vi "Alarm Editor.vi"() -> ()   [LabVIEW 2020]
uses:
  <vilib>/Tag Engine/Tag Expr/Tag Expr.lvclass
  C:/Program Files (x86)/National Instruments/LabVIEW 2020/vi.lib/LAVA/muParser/mupExpr/mupExpr.lvclass
  <vilib>/Tag Engine/Tag/Tag.lvclass/Tag.ctl
  cd2f347f-65b6-438d-b97c-e7d356f4cfc3.vi
  <vilib>/Tag Engine/API/Get Tag Value_ByRef.vi
  <vilib>/Tag Engine/API/Get Tag.vi
  <vilib>/Tag Engine/API/Send Tag SetRequest_ByRef.vi
  <vilib>/Tag Engine/Tag/Read Value.vi
  <vilib>/Tag Engine/Tag/Read Timestamp.vi
  <vilib>/Tag Engine/Tag/Write SetRequest.vi
  <vilib>/Tag Engine/Core/Tag Lookup_By Name.vi
  c6dfc7c3-9080-4d04-b6fb-254d10b3aea1.vi
panel:
  in  "Cancel":bool
  in  "OK":bool
  out "Name2":string
  out "Valid2":bool
  in  "Condition2":string
  out "Name1":string
  out "Valid1":bool
  in  "Condition1":string
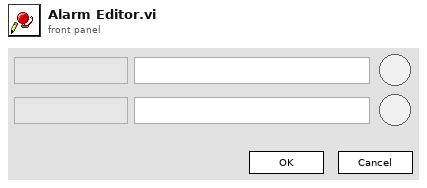
[diagram p1: front panel]
types:
  T1 = cluster{"Alarms":cluster{"Name":string, "Condition":string}[]}
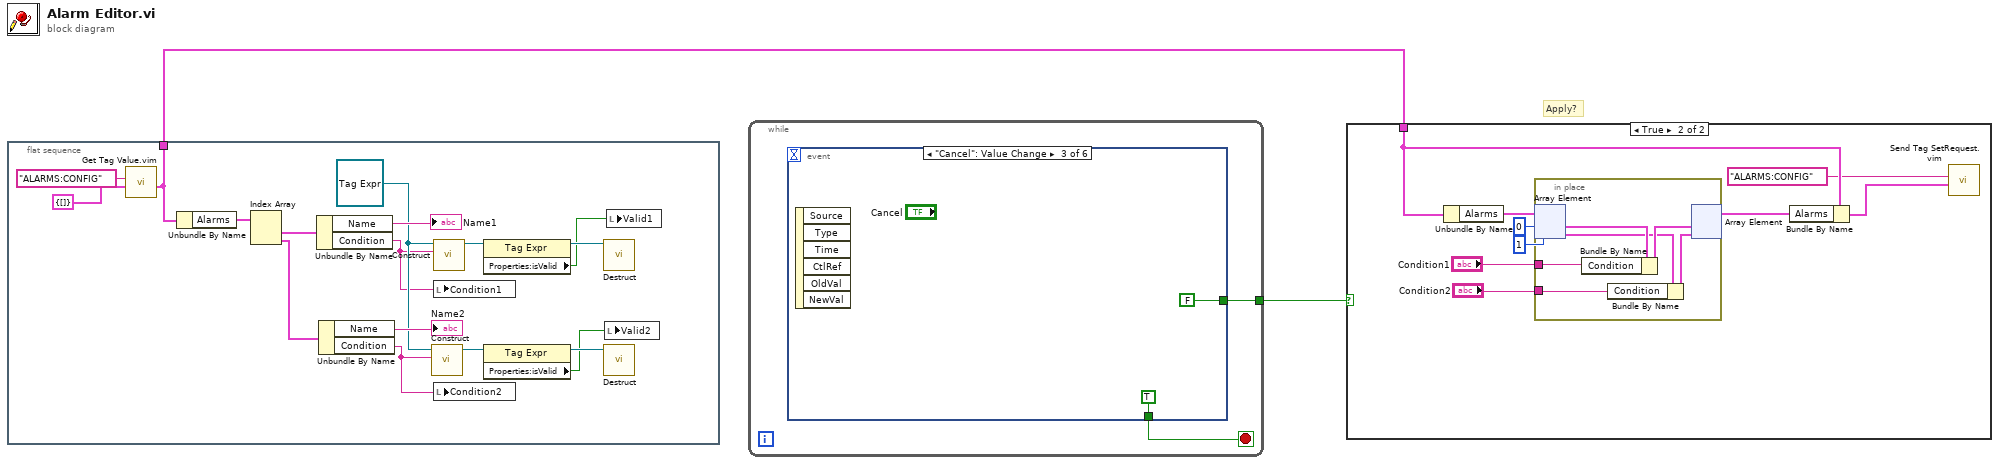
[diagram p0: block diagram]
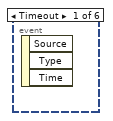
[diagram p3: hidden frame]
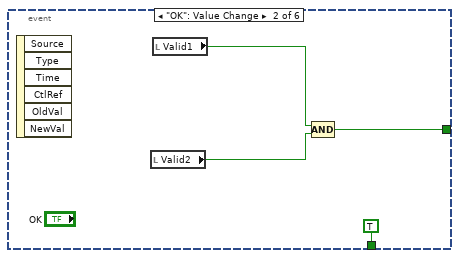
[diagram p4: hidden frame]
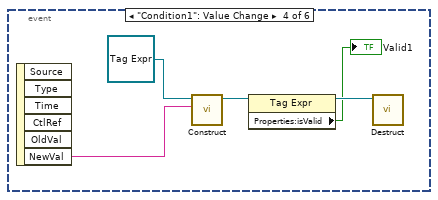
[diagram p5: hidden frame]
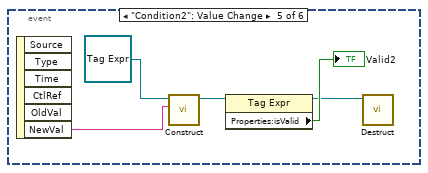
[diagram p6: hidden frame]
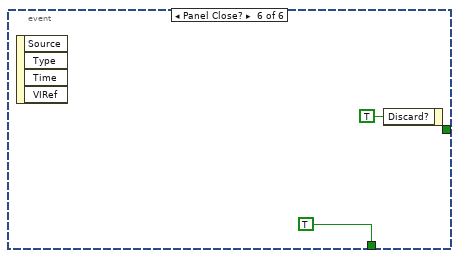
[diagram p7: hidden frame]
diagram:
  # "Apply?"
  n1 = flat-sequence {
    tunnel: [w3] -> w1
    frame #0 {
      w12 = refnum<class "Tag Expr.lvclass"> refnum ("Tag Expr in")
      n2 = call "Get Tag Value.vim"("Default (Void)"=T1 {"Alarms"=[]} ("Config"), "Tag Name(s)/Ref(s)"="ALARMS:CONFIG") -> ("Value(s)"=w3:T1)  [unwired: 6 in, 3 out]
      n3 = Unbundle By Name(w3) -> ("Alarms"=w17:cluster{"Name":string, "Condition":string}[])
      n4 = Index Array(array=w17) -> (element #1=w16:cluster{"Name":string, "Condition":string}, element #2=w14:cluster{"Name":string, "Condition":string})  [unwired: 2 in]
      n5 = Unbundle By Name(w16) -> ("Name"=→"Name1":string, "Condition"=w4:string)
      n6 = Unbundle By Name(w14) -> ("Name"=→"Name2":string, "Condition"=w5:string)
      n7 = call-dynamic "Construct.vi"("Expression"=w5, "Tag Expr in"=w12) -> ("Tag Expr out"=w10:refnum<class "Tag Expr.lvclass">)  [unwired: 6 in, 3 out]
      n8 = call-dynamic "Construct.vi"("Expression"=w4, "Tag Expr in"=w12) -> ("Tag Expr out"=w11:refnum<class "Tag Expr.lvclass">)  [unwired: 6 in, 3 out]
      n9 = local write "Condition1"(w4) -> ()
      n10 = local write "Condition2"(w5) -> ()
      n11 = property class="Tag Expr"(reference=w11) -> (reference out=w9:refnum<class "Tag Expr.lvclass">, "Properties:isValid"=w7:bool)  [unwired: 1 in, 1 out]
      n12 = property class="Tag Expr"(reference=w10) -> (reference out=w8:refnum<class "Tag Expr.lvclass">, "Properties:isValid"=w6:bool)  [unwired: 1 in, 1 out]
      n13 = call-dynamic "Destruct.vi"("muExpr in"=w9) -> ()  [unwired: 10 in, 1 out]
      n14 = call-dynamic "Destruct.vi"("muExpr in"=w8) -> ()  [unwired: 10 in, 1 out]
      n15 = local write "Valid2"(w6) -> ()
      n16 = local write "Valid1"(w7) -> ()
    }
  }
  n17 = while {
    tunnel: [w20] -> w2
    stop <- w21 stop-if-true
    n18 = event shown="[2] \"Cancel\": Value Change" {
      selector: _ -> [_ _ _ _ _ _]
      dyn-events: _ -> [_ _ _ _ _ _]
      timeout: _ -> [_ _ _ _ _ _]
      tunnel: [_ TRUE TRUE _ _ TRUE] -> w21
      tunnel: [_ w23 FALSE _ _ _] -> w20
      event Timeout {
        n19 = event-data() -> ()  [unwired: 1 in, 3 out]
      }
      event "OK": Value Change {
        n20 = event-data() -> ()  [unwired: 1 in, 6 out]
        n21 = local read "Valid2"() -> (w24:bool)
        n22 = local read "Valid1"() -> (w25:bool)
        n23 = Compound Arithmetic op=AND(w25, w24) -> (w23:bool)
      }
      event "Cancel": Value Change {
        n24 = event-data() -> ()  [unwired: 1 in, 6 out]
      }
      event "Condition1": Value Change {
        n25 = event-data() -> ("NewVal"=w31:string)  [unwired: 1 in, 5 out]
        n26 = call-dynamic "Construct.vi"("Expression"=w31, "Tag Expr in"=refnum<class "Tag Expr.lvclass"> refnum) -> ("Tag Expr out"=w30:refnum<class "Tag Expr.lvclass">)  [unwired: 6 in, 3 out]
        n27 = property class="Tag Expr"(reference=w30) -> (reference out=w29:refnum<class "Tag Expr.lvclass">, "Properties:isValid"=→"Valid1":bool)  [unwired: 1 in, 1 out]
        n28 = call-dynamic "Destruct.vi"("muExpr in"=w29) -> ()  [unwired: 10 in, 1 out]
      }
      event "Condition2": Value Change {
        n29 = event-data() -> ("NewVal"=w35:string)  [unwired: 1 in, 5 out]
        n30 = call-dynamic "Construct.vi"("Expression"=w35, "Tag Expr in"=refnum<class "Tag Expr.lvclass"> refnum) -> ("Tag Expr out"=w36:refnum<class "Tag Expr.lvclass">)  [unwired: 6 in, 3 out]
        n31 = property class="Tag Expr"(reference=w36) -> (reference out=w33:refnum<class "Tag Expr.lvclass">, "Properties:isValid"=→"Valid2":bool)  [unwired: 1 in, 1 out]
        n32 = call-dynamic "Destruct.vi"("muExpr in"=w33) -> ()  [unwired: 10 in, 1 out]
      }
      event Panel Close? {
        n33 = event-data() -> ()  [unwired: 1 in, 4 out]
        n34 = event-data("Discard?"=TRUE) -> ()  [unwired: 1 in, 1 out]
      }
    }
  }
  n35 = case shown="True" w2 {
    tunnel: w1 -> [_ w47]
    frame False {
    }
    frame True {
      n36 = Unbundle By Name(w47) -> ("Alarms"=w48:cluster{"Name":string, "Condition":string}[])
      n37 = in-place {
        in-place-border: "Condition1" -> [w50]
        in-place-border: "Condition2" -> [w49]
        n38 = in-place-array #1(w48, 0, 1) -> (w54:cluster{"Name":string, "Condition":string}, w52:cluster{"Name":string, "Condition":string})
        n39 = Bundle By Name(cluster=w54, "Condition"=w50) -> (w53:cluster{"Name":string, "Condition":string})
        n40 = Bundle By Name(cluster=w52, "Condition"=w49) -> (w51:cluster{"Name":string, "Condition":string})
        n41 = in-place-array #1(w53, w51) -> (w46:cluster{"Name":string, "Condition":string}[])  [unwired: 2 out]
      }
      n42 = Bundle By Name(cluster=w47, "Alarms"=w46) -> (w40:T1)
      n43 = call "Send Tag SetRequest.vim"("Value"=w40, "Tag Name(s)/Ref(s)"="ALARMS:CONFIG") -> ()  [unwired: 7 in, 3 out]
    }
  }
